vi "Filter Item.vi"(6 "Case Sensitive?":bool, 7 "Filter Type":T1, 8 "error in (no error)":errorcluster, 9 "Filter Value":string, 10 "Filter Column":T2, 11 "Item in":refnum<class "Item.lvclass">) -> (0 "error out":errorcluster, 2 "Include?":bool, 3 "Item out":refnum<class "Item.lvclass">)   [LabVIEW 2020, in "VI Properties Editor.lvlib" / "Item.lvclass"]
doc: "Checks whether <B>Item in</B> will be included in a filter defined by the other inputs."
uses:
  Item.lvclass
  CTLs/Filter Column.ctl
  CTLs/Filter Type.ctl
  VI Properties Editor.lvlib
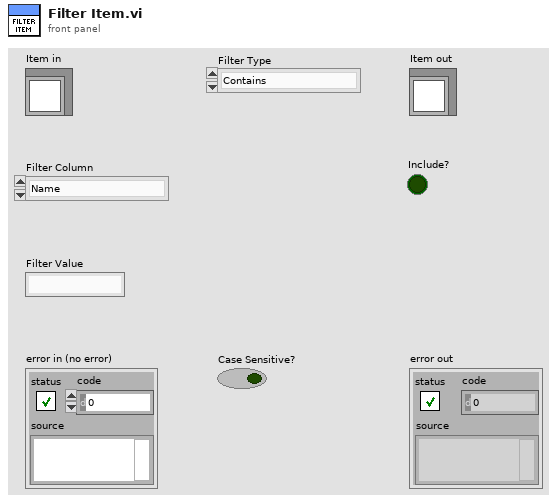
[diagram p1: front panel]
types:
  T1 = typedef "VI Properties Editor.lvlib/Filter Type.ctl" = enum16{"Contains", "Equals", "Starts with", "Ends with", "Is empty", "Does not contain", "Does not equal", "Is not empty"}
  T2 = typedef "VI Properties Editor.lvlib/Filter Column.ctl" = enum16{"Name", "Path", "Type", "Window Title", "Description", "Help Path", "Help Tag", "Custom Title?", "Reentrancy", "Inlined?", "Help URL", "Help Type", "Allow Debugging?", "Auto Error Handling?", "Run When Opened?", "Suspend When Called?", "Priority", "Preferred Exec Sytem", "Control Label", "Control Caption", "Control Description", "Control Tip Strip"}
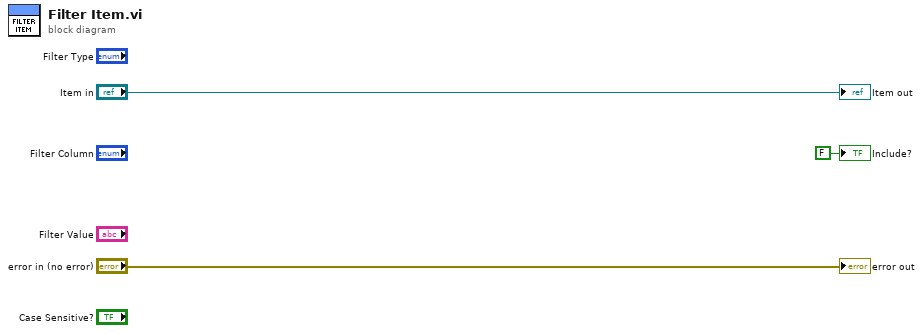
[diagram p0: block diagram]
diagram:
  "error out" <- "error in (no error)"
  "Item out" <- "Item in"
  "Include?" <- FALSE ("Include?")
